vi "Write TKEEP Core.vi"(10 "value":bool[](array[boolean]), 11 "niInstr AXI4-Stream Writer FXP32x1 v1 FPGA in":refnum<class "niInstr AXI4-Stream Writer FXP32x1 v1 FPGA.lvclass">) -> (3 "niInstr AXI4-Stream Writer FXP32x1 v1 FPGA out":refnum<class "niInstr AXI4-Stream Writer FXP32x1 v1 FPGA.lvclass">)   [LabVIEW 2015, in "niInstr AXI4-Stream Writer FXP32x1 v1 FPGA.lvclass"]
uses:
  <instrlib>/_niInstr/CLIP Adapters/v1/FPGA/AXI4-Stream/Writer FXP32x1/niInstr AXI4-Stream Writer FXP32x1 v1 FPGA.lvclass
  <instrlib>/_niInstr/CLIP Adapters/v1/FPGA/AXI4-Stream/Writer FXP32x1/niInstr AXI4-Stream Writer FXP32x1 v1 FPGA.lvclass/niInstr AXI4-Stream Writer FXP32x1 v1 FPGA.ctl
  <vilib>/rvi/eio/common/nirviEmuTemplateMethod_errors.vi
  <vilib>/eio/EIONode/EIONode.xnode
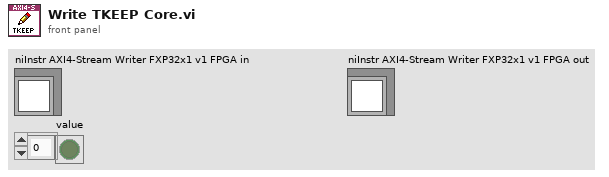
[diagram p1: front panel]
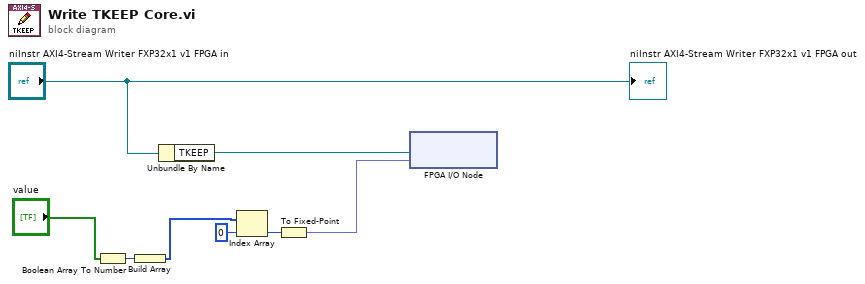
[diagram p0: block diagram]
diagram:
  n1 = Boolean Array To Number(Boolean array="value") -> (number=w2:u32)
  n2 = Build Array(w2) -> (w1:u32[])
  n3 = Unbundle By Name("niInstr AXI4-Stream Writer FXP32x1 v1 FPGA in") -> ("TKEEP"=w4:refnum<k21>)
  n4 = Index Array(array=w1, index=0) -> (element=w6:u32)
  n5 = To Fixed-Point(number=w6) -> (fixed-point=w5:fxp<+,4,4>)  [unwired: 1 in]
  n6 = xnode "FPGA I/O Node"("I/O Item"=w5, "FPGA I/O In"=w4) -> ()  [unwired: 1 out]
  "niInstr AXI4-Stream Writer FXP32x1 v1 FPGA out" <- "niInstr AXI4-Stream Writer FXP32x1 v1 FPGA in"
